vi "Omron TCP FINS-Write Data(Boolean Array).vi"(8 "error in":errorcluster, 9 "Data":bool[](array[boolean]), 10 "Write Setting(Boolean Array)":T1={"I/O Memory Address"=130, "Data Address"=0} {"I/O Memory Address" items=["DM"=130, "CIO"=176, "WR"=177, "HR"=178, "AR"=179, "TIM"=137, "EM"=152]}, 11 "Buffer Data In":T2) -> (0 "error out":errorcluster, 3 "Buffer Data Out":T2)   [LabVIEW 2016]
uses:
  Data Def/Omron TCP FINS-Buffer Data.ctl
  Data Def/Omron TCP FINS-Command Code.ctl
  Data Def/Omron TCP FINS-FINS Command Frame.ctl
  Data Def/Omron TCP FINS-Memory Area Write Data.ctl
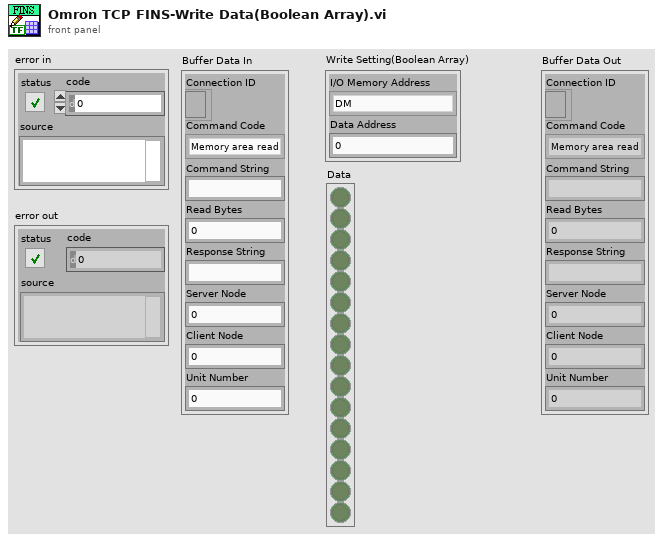
[diagram p1: front panel]
types:
  T1 = cluster{"I/O Memory Address":u8, "Data Address":u16}
  T2 = typedef "Omron TCP FINS-Buffer Data.ctl" = cluster{"Connection ID":refnum<k5>, "Command Code":T3, "Command String":string, "Read Bytes":i32, "Response String":string, "Server Node":u8, "Client Node":u8, "Unit Number":u8}
  T3 = typedef "Omron TCP FINS-Command Code.ctl" = enum16{"Memory area read", "Memory area write"}
  T4 = typedef "Omron TCP FINS-Memory Area Write Data.ctl" = cluster{"I/O Memory Address":u8, "Beginning Address":u16, "Data":i16[]}
  T5 = typedef "Omron TCP FINS-FINS Command Frame.ctl" = cluster{"Command Code":T3, "Command Data":variant}
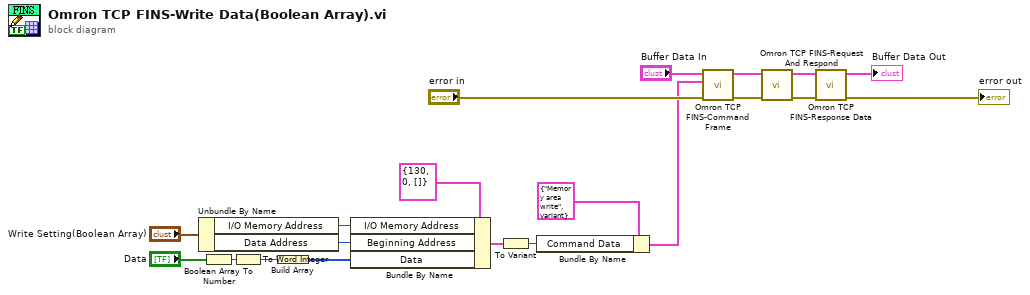
[diagram p0: block diagram]
diagram:
  n1 = Unbundle By Name("Write Setting(Boolean Array)") -> ("I/O Memory Address"=w7:u8, "Data Address"=w6:u16)
  n2 = Boolean Array To Number(Boolean array="Data") -> (number=w3:u32)
  n3 = To Word Integer(number=w3) -> (16bit integer=w2:i16)
  n4 = Build Array(w2) -> (w1:i16[])
  n5 = Bundle By Name(cluster=T4 {"I/O Memory Address"=130, "Beginning Address"=0, "Data"=[]} ("Memory Area Write Data"), "I/O Memory Address"=w7, "Beginning Address"=w6, "Data"=w1) -> (w9:T4)
  n6 = To Variant(anything=w9) -> (Variant=w18:variant)
  n7 = Bundle By Name(cluster=T5 {"Command Code"=enum."Memory area write", "Command Data"=variant} ("FINS Command Frame"), "Command Data"=w18) -> (w16:T5)
  n8 = call "Omron TCP FINS-Command Frame.vi"("error in"="error in", "FINS Command Frame"=w16, "Buffer Data In"="Buffer Data In") -> ("error out"=w14:errorcluster, "Buffer Data Out"=w15:T2)  [unwired: 7 in]
  n9 = call "Omron TCP FINS-Request And Respond.vi"("error in"=w14, "Buffer Data In"=w15) -> ("error out"=w12:errorcluster, "Buffer Data Out"=w13:T2)  [unwired: 8 in]
  n10 = call "Omron TCP FINS-Response Data.vi"("error in"=w12, "Buffer Data In"=w13) -> ("error out"=→"error out":errorcluster, "Buffer Data Out"=→"Buffer Data Out":T2)  [unwired: 7 in, 1 out]
